vi "Reformat LV Version String.vi"(11 "Version String (2014)":string) -> (3 "Short Version String (14.0)":string)   [LabVIEW 2014, in "lv-build-library.lvlib"]
uses:
  lv-build-library.lvlib
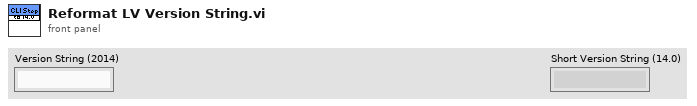
[diagram p1: front panel]
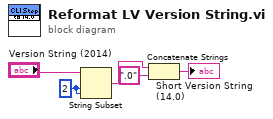
[diagram p0: block diagram]
diagram:
  w2 = 2 ("offset (0)")
  n1 = String Subset(string="Version String (2014)", offset (0)=w2, length (rest)=w2) -> (substring=w3:string)
  n2 = Concatenate Strings(w3, ".0" ("string")) -> (→"Short Version String (14.0)":string)
